vi "videos.list.vi"(8 "error in":errorcluster, 11 "asset in":refnum<class "asset.lvclass">) -> (0 "error out":errorcluster, 2 "videos":map{string, string}(c390), 3 "asset out":refnum<class "asset.lvclass">)   [LabVIEW 2020, in "asset.lvclass"]
uses:
  asset.lvclass
  asset.lvclass/asset.ctl
  nominal types/dataScope/type.ctl
  datascopes.get.vi
  nominal types/dataScope/dataScopes.lvlib
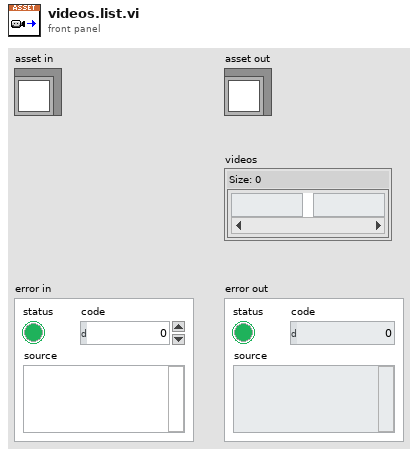
[diagram p1: front panel]
types:
  T1 = typedef "dataScopes.lvlib/data_scopes.ctl" = T2[]
  T2 = typedef "dataScopes.lvlib/data_scope.ctl" = cluster{"dataScopeName":string, "dataSource":T3, "seriesTags":map{string, string}, "offset":T5}
  T3 = typedef "dataScopes.lvlib/data_source.ctl" = cluster{"type":T4, "rid":string}
  T4 = typedef "dataScopes.lvlib/type.ctl" = enum16{"dataset", "connection", "logSet", "video"}
  T5 = typedef "dataScopes.lvlib/offset.ctl" = cluster{"seconds":i32, "nanos":i32, "picos":i32}
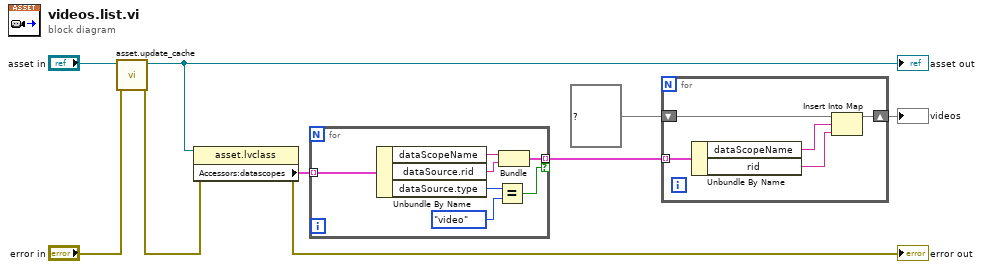
[diagram p0: block diagram]
diagram:
  n1 = call "asset.update_cache.vi"("error in"="error in", "asset in"="asset in") -> ("error out"=w4:errorcluster, "asset out"=w6:refnum<class "asset.lvclass">)  [unwired: 8 in]
  "asset out" <- w6
  n2 = property class="asset.lvclass"(reference=w6, error in=w4) -> (error out=→"error out":errorcluster, "Accessors:datascopes"=w9:T1)  [unwired: 1 out]
  n3 = for {
    tunnel: w9 -> [w14] mode=indexing
    tunnel: [w10] -> w3 mode=indexing if=w13
    n4 = Unbundle By Name(w14) -> ("dataScopeName"=w11:string, "dataSource.rid"=w12:string, "dataSource.type"=w16:T4)
    n5 = Equal?(x=w16, y=type."video") -> (x = y?=w13:bool)
    n6 = Bundle("dataScopeName"=w11, "rid"=w12) -> (w10:cluster{"dataScopeName":string, "rid":string})  [unwired: 1 in]
  }
  n7 = for {
    tunnel: w3 -> [w21] mode=indexing
    shift-right: [w17] -> w1
    shift-left: map{string, string} {} ("map in") -> [w18]
    n8 = Unbundle By Name(w21) -> ("dataScopeName"=w20:string, "rid"=w19:string)
    n9 = Insert Into Map(map in=w18, key=w20, value=w19) -> (map out=w17:map{string, string})  [unwired: 2 out]
  }
  "videos" <- w1
